vi "init.vi"(8 "error in (no error)":errorcluster, 9 "SwapBytes":bool, 10 "Size":i32, 11 "U8ArrayBuilderAutoIndexing in":refnum<class "U8ArrayBuilderAutoIndexing.lvclass">) -> (0 "error out":errorcluster, 3 "U8ArrayBuilderAutoIndexing out":refnum<class "U8ArrayBuilderAutoIndexing.lvclass">)   [LabVIEW 2016, in "RTUtilities.lvlib" / "U8ArrayBuilderAutoIndexing.lvclass"]
uses:
  U8ArrayBuilderAutoIndexing.lvclass
  U8ArrayBuilderManualIndexing/U8ArrayBuilderManualIndexing.lvclass
  U8ArrayBuilderAutoIndexing.lvclass/U8ArrayBuilderAutoIndexing.ctl
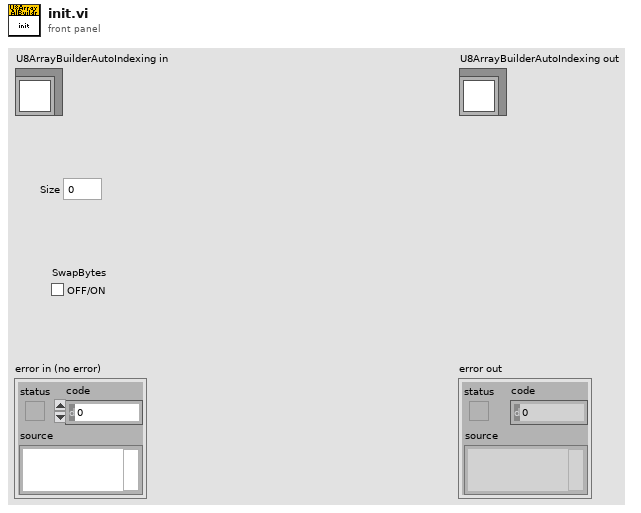
[diagram p1: front panel]
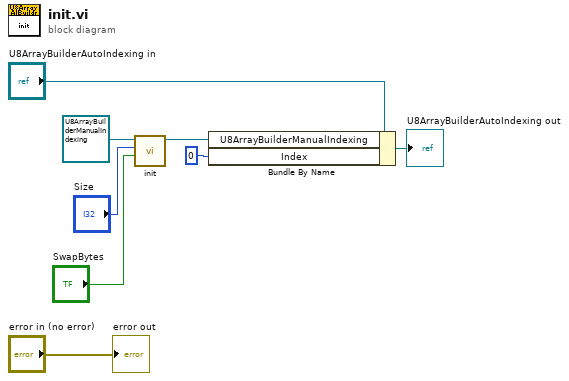
[diagram p0: block diagram]
diagram:
  n1 = call "init.vi"("SwapBytes"="SwapBytes", "Size"="Size", "U8ArrayBuilderManualIndexing in"=refnum<class "U8ArrayBuilderManualIndexing.lvclass"> refnum ("RTUtilities.lvlib:U8ArrayBuilderManualIndexing.lvclass")) -> ("U8ArrayBuilderManualIndexing out"=w1:refnum<class "U8ArrayBuilderManualIndexing.lvclass">)  [unwired: 7 in, 1 out]
  n2 = Bundle By Name(cluster="U8ArrayBuilderAutoIndexing in", "U8ArrayBuilderManualIndexing"=w1, "Index"=0) -> (→"U8ArrayBuilderAutoIndexing out":refnum<class "U8ArrayBuilderAutoIndexing.lvclass">)
  "error out" <- "error in (no error)"
